vi "OAT Even Angle Signal Sample Rate Conversion (1 Channel).vi"(0 "even-angle signal":cluster{"r0":dbl, "dr":dbl, "Y":dbl[]}={"r0"=0.0, "dr"=1.0, "Y"=[]} {"r0" format="%.2p"; "dr" format="%.2p"; "Y" format="%.2f"}, 2 "reset? (F)":bool, 5 "even-angle channel info":T3={"channel name"="", "description"="", " channel info"={"sensor sensitivity"=1000.0, "engineering units"=1, "dB reference"=1.0, "custom label"="EU", "weighting filter"=0, "pregain"=0.0}} {"channel info"."pregain" format="%.2f"; "channel info"."weighting filter" items=["Linear", "A-weighting", "B-weighting", "C-weighting", "ITU-R 468-4", "Dolby", "CCITT", "C-message", "Wb", "Wc", "Wd", "We", "Wf", "Wh", "Wj", "Wk", "Wm", "AES17 20 kHz lowpass", "AES17 40 kHz lowpass", "AES17 20 kHz highpass", "AES17 40 kHz highpass"]; "channel info"."dB reference" format="%^.1e"; "channel info"."engineering units" items=["custom..."=0, "V"=1, "A"=21, "C"=30, "pC"=31, "s"=32, "-"=29, "Pa"=2, "N"=20, "g"=3, "m/s^2"=4, "m/s"=5, "m"=6, "mm/s"=12, "mm"=13, "micron/s"=14, "micron"=15, "in/s^2"=7, "in/s"=8, "in"=9, "mil/s"=10, "mil"=11, "rad/s^2"=16, "rad/s"=17, "rad"=18, "deg/s^2"=26, "deg/s"=27, "deg"=28, "RPM"=22, "cycle/s^2"=23, "Hz"=24, "cycle"=25, "strain"=19]; "channel info"."sensor sensitivity" format="%#_5f"}, 7 "even-angle position info":T2, 9 "new dr":dbl=1.0 format="%.2p", 11 "error in (no error)":errorcluster, 12 "interpolation mode":u16(ring)=1 items=["coerce", "linear", "spline", "FIR filter"], 13 "FIR filter specifications":T1={"alias rejection [dB]"=120.0, "normalized bandwidth"=0.4536} {"normalized bandwidth" format="%.4f"; "alias rejection [dB]" format="%.2f"}) -> (4 "even-angle signal out":cluster{"r0":dbl, "dr":dbl, "Y":dbl[]}={"r0"=0.0, "dr"=1.0, "Y"=[]} {"r0" format="%.2p"; "dr" format="%.2p"; "Y" format="%.2f"}, 6 "even-angle channel info out":T3={"channel name"="", "description"="", " channel info"={"sensor sensitivity"=1000.0, "engineering units"=1, "dB reference"=1.0, "custom label"="EU", "weighting filter"=0, "pregain"=0.0}} {"channel info"."pregain" format="%.2f"; "channel info"."weighting filter" items=["Linear", "A-weighting", "B-weighting", "C-weighting", "ITU-R 468-4", "Dolby", "CCITT", "C-message", "Wb", "Wc", "Wd", "We", "Wf", "Wh", "Wj", "Wk", "Wm", "AES17 20 kHz lowpass", "AES17 40 kHz lowpass", "AES17 20 kHz highpass", "AES17 40 kHz highpass"]; "channel info"."dB reference" format="%^.1e"; "channel info"."engineering units" items=["custom..."=0, "V"=1, "A"=21, "C"=30, "pC"=31, "s"=32, "-"=29, "Pa"=2, "N"=20, "g"=3, "m/s^2"=4, "m/s"=5, "m"=6, "mm/s"=12, "mm"=13, "micron/s"=14, "micron"=15, "in/s^2"=7, "in/s"=8, "in"=9, "mil/s"=10, "mil"=11, "rad/s^2"=16, "rad/s"=17, "rad"=18, "deg/s^2"=26, "deg/s"=27, "deg"=28, "RPM"=22, "cycle/s^2"=23, "Hz"=24, "cycle"=25, "strain"=19]; "channel info"."sensor sensitivity" format="%#_5f"}, 8 "even-angle position info out":T2, 15 "error out":errorcluster)   [LabVIEW 2017, in "SoundVib_OAUtility.lvlib"]
doc: "Converts the sample rate of the even-angle signal. Use this VI to specify a new revolution interval for sampling. Each instance of this VI maintains its own state; use the N waveforms instance of this VI to process an array of channels. Wire data to the <B>even-angle signal</B> input to determine the polymorphic instance to use or manually select the instance."
uses:
  <vilib>/addons/Sound and Vibration/Order Analysis/Utility/SoundVib_OAUtility.lvlib
  <vilib>/addons/_NISVFA/_Shared subVIs/Controls/svc_Resampled Channel Info.ctl
  <vilib>/addons/_NISVFA/_Shared subVIs/Controls/svc_Channel Info.ctl
  <vilib>/addons/_NISVFA/_Shared subVIs/Controls/svc_Engineering Units Text Ring.ctl
  <vilib>/addons/_NISVFA/_Shared subVIs/Controls/svc_Weighting Filter Text Ring.ctl
  <vilib>/addons/Sound and Vibration/Order Analysis/Misc/OAT Position Info.ctl
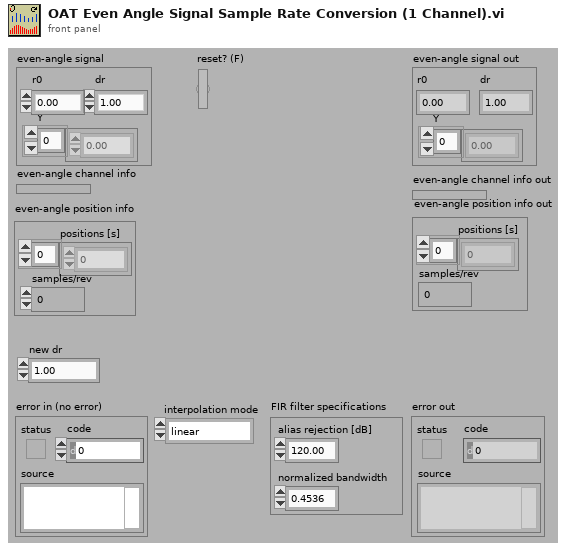
[diagram p1: front panel]
types:
  T1 = cluster{"alias rejection [dB]":dbl, "normalized bandwidth":dbl}
  T2 = typedef "OAT Position Info.ctl" = cluster{"positions [s]":dbl[], "samples/rev":dbl}
  T3 = typedef "svc_Resampled Channel Info.ctl" = cluster{"channel name":string, "description":string, " channel info":T4}
  T4 = typedef "svc_Channel Info.ctl" = cluster{"sensor sensitivity":dbl, "engineering units":T5, "dB reference":dbl, "custom label":string, "weighting filter":T6, "pregain":dbl}
  T5 = typedef "svc_Engineering Units Text Ring.ctl" = u16
  T6 = typedef "svc_Weighting Filter Text Ring.ctl" = u16
  T7 = cluster{"alias rejection (dB)":dbl, "normalized bandwidth":dbl}
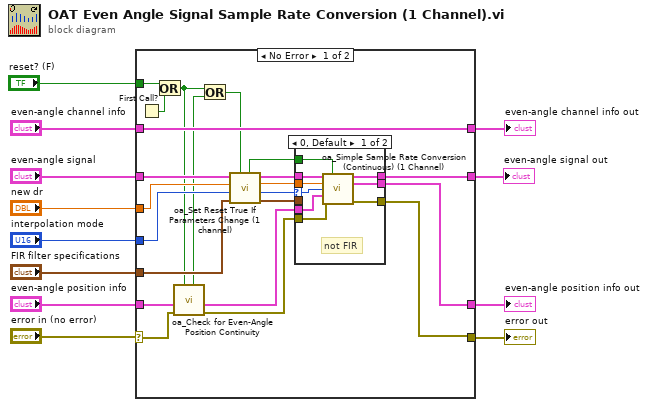
[diagram p0: block diagram]
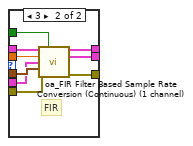
[diagram p2: hidden frame]
diagram:
  n1 = case shown="No Error" "error in (no error)" {
    selector: "error in (no error)" -> [w14 w53]
    tunnel: "even-angle signal" -> [w33 w56]
    tunnel: "new dr" -> [w30 _]
    tunnel: "interpolation mode" -> [w34 _]
    tunnel: "FIR filter specifications" -> [w29 _]
    tunnel: [w23 w56] -> w8
    tunnel: [w21 w53] -> w6
    tunnel: "even-angle channel info" -> [w20 w55]
    tunnel: [w20 w55] -> w3
    tunnel: "even-angle position info" -> [w24 w54]
    tunnel: [w22 w54] -> w2
    tunnel: "reset? (F)" -> [w32 _]
    frame No Error {
      n2 = First Call?() -> (First Call?: T/F=w31:bool)
      n3 = Or(x=w32, y=w31) -> (x .or. y?=w17:bool)
      n4 = call <vilib>:"oa_Check for Even-Angle Position Continuity.vi"("reset in"=w17, "error in (no error)"=w14, "even-angle position info"=w24) -> ("error out"=w13:errorcluster, "even-angle position info dup"=w18:T2, "position not continuous"=w15:bool)  [unwired: 6 in]
      n5 = Or(x=w17, y=w15) -> (x .or. y?=w16:bool)
      n6 = call <vilib>:"oa_Set Reset True If Parameters Change (1 channel).vi"("reset? (T) in"=w16, "FIR filter specifications in"=w29, "interpolation mode in"=w34, "dr in"=w30, "even angle signal in"=w33) -> ("FIR filter specifications out"=w19:T7, "interpolation mode out"=w25:u16, "dr out"=w26:dbl, "even angle signal out"=w28:cluster{"r0":dbl, "dr":dbl, "Y":dbl[]}, "reset? (T) out"=w27:bool)  [unwired: 2 in]
      n7 = case shown="0, Default" w25 {
        selector: w25 -> [w36 _]
        tunnel: w28 -> [w43 w52]
        tunnel: w27 -> [w42 w45]
        tunnel: w26 -> [w41 w51]
        tunnel: w18 -> [w40 w49]
        tunnel: [w39 w48] -> w23
        tunnel: [w38 w47] -> w22
        tunnel: [w37 w46] -> w21
        tunnel: w19 -> [_ w50]
        tunnel: w13 -> [w35 w44]
        frame 0, Default {
          # "not FIR"
          n8 = call <vilib>:"oa_Simple Sample Rate Conversion (Continuous) (1 Channel).vi"("even angle signal in"=w43, "reset? (T)"=w42, "dr"=w41, "interpolation mode"=w36, "even angle position info"=w40, "error in (no error)"=w35) -> ("even angle signal out"=w39:cluster{"r0":dbl, "dr":dbl, "Y":dbl[]}, "out even angle position info"=w38:T2, "error out"=w37:errorcluster)  [unwired: 7 in]
        }
        frame 3 {
          # "FIR"
          n9 = call <vilib>:"oa_FIR Filter Based Sample Rate Conversion (Continuous) (1 channel).vi"("even angle signal in"=w52, "reset? (T)"=w45, "dr"=w51, "even angle position info"=w49, "FIR filter specifications"=w50, "error in (no error)"=w44) -> ("even angle signal out"=w48:cluster{"r0":dbl, "dr":dbl, "Y":dbl[]}, "even angle position info out"=w47:T2, "error out"=w46:errorcluster)  [unwired: 7 in]
        }
      }
    }
    frame Error {
    }
  }
  "error out" <- w6
  "even-angle signal out" <- w8
  "even-angle channel info out" <- w3
  "even-angle position info out" <- w2
